vi "Command Started.vi"(8 "error in (no error)":errorcluster, 10 "Command Name (Instance)":string, 11 "Starting Command in":refnum<class "Starting Command.lvclass">) -> (0 "error out":errorcluster, 3 "Starting Command out":refnum<class "Starting Command.lvclass">)   [LabVIEW 2014, in "Robot Actor Framework.lvlib" / "Command Processor Actor.lvlib" / "Starting Command.lvclass"]
uses:
  Starting Command.lvclass
  <vilib>/ActorFramework/Message Enqueuer/Message Priority.ctl
  <vilib>/ActorFramework/Actor/Actor.lvclass/Actor.ctl
  <vilib>/ActorFramework/Message Enqueuer/Message Enqueuer.lvclass/Message Enqueuer.ctl
  <vilib>/ActorFramework/Message Enqueuer/Init from Existing Queue.vi
  <vilib>/ActorFramework/Message Enqueuer/Enqueue.vi
  <vilib>/ActorFramework/Message Priority Queue/Priority Enqueue.vi
  Command Processor Actor Class/Command Processor Actor.lvclass
  <vilib>/ActorFramework/Message Enqueuer/Message Enqueuer.lvclass
  Command Processor Actor Messages/Go To Running Command Msg/Go To Running Command Msg.lvclass
  <vilib>/ActorFramework/Actor/Actor.lvclass
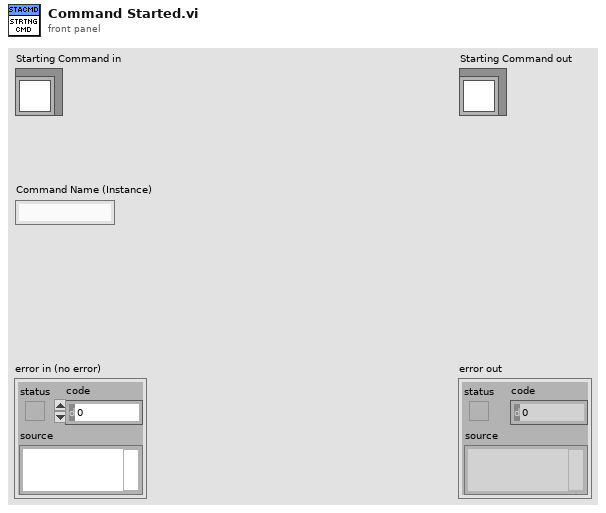
[diagram p1: front panel]
types:
  T1 = typedef "Actor Framework.lvlib/Message Enqueuer.lvclass/Message Priority.ctl" = enum16{"Low", "Normal", "High"}
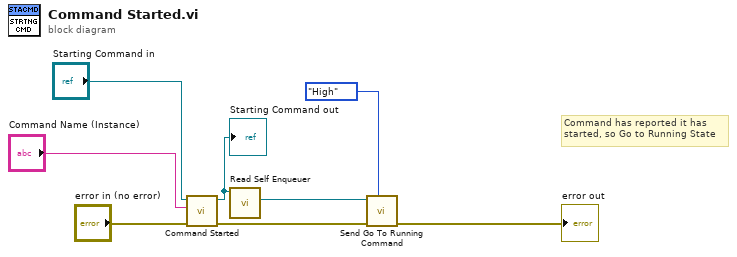
[diagram p0: block diagram]
diagram:
  # "Command has reported it has \nstarted, so Go to Running State"
  n1 = call-parent "Command Started.vi"("error in (no error)"="error in (no error)", "Command Name (Instance)"="Command Name (Instance)", "Command Processor Actor in"="Starting Command in") -> ("error out"=w4:errorcluster, "Command Processor Actor out"=w5:refnum<class "Starting Command.lvclass">)  [unwired: 7 in]
  "Starting Command out" <- w5
  n2 = call <vilib>:"Read Self Enqueuer.vi"("Actor"=w5) -> ("Self Enqueuer"=w8:refnum<class "Message Enqueuer.lvclass">)  [unwired: 10 in]
  n3 = call "Send Go To Running Command.vi"("Message Priority (Normal)"=Message_Priority."High", "error in (no error)"=w4, "Message Enqueuer"=w8) -> ("error out"=→"error out":errorcluster)  [unwired: 7 in, 1 out]
